vi "ROV Control via UDP Protocole. upgrade.vi"() -> ()   [LabVIEW 2012]
uses:
  <vilib>/Utility/inputDevices.llb/closeJoystick.vi
  <vilib>/Utility/inputDevices.llb/joystickAcquire.vi
panel:
  in  "J":dbl
  out "CASE Z R":u32
  out "CASE UP AND DOWN":u32
  in  "LED STATE":dbl
  in  "N result":string
  out "CASE MOTION":u32
  out "Y O":dbl
  out "U O":dbl
  out "Z O":dbl
  out "X O":dbl
  out "Z R O":dbl
  out "axis info":T1
  out "direction info":T2
  out "button info":T3
  in  "device index":i32
  out "joystick info":T4(array[cluster])
  out "Result":string
  in  "I":dbl
  in  "H":dbl
  in  "G":dbl
  in  "D":dbl
  in  "E":dbl
  in  "Z":dbl
  in  "F":dbl
  in  "C":dbl
  in  "Y":dbl
  in  "B":dbl
  in  "A":dbl
  in  "?":bool
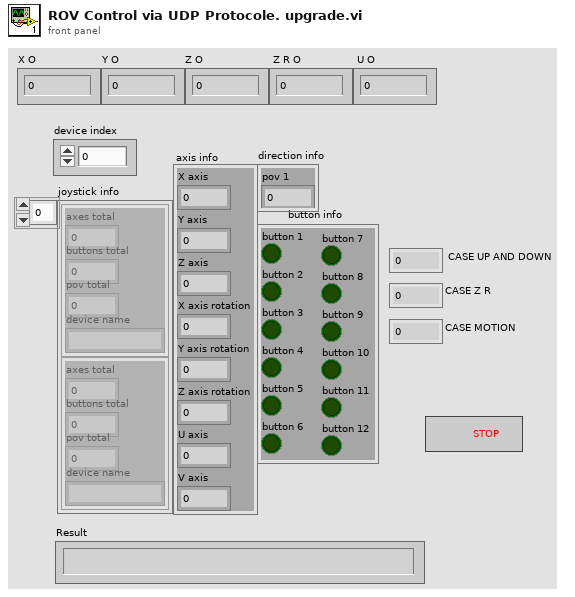
[diagram p1: front panel]
types:
  T1 = cluster{"X axis":i32, "Y axis":i32, "Z axis":i32, "X axis rotation":i32, "Y axis rotation":i32, "Z axis rotation":i32, "U axis":i32, "V axis":i32}
  T2 = cluster{"pov 1":i32, "pov 2":i32, "pov 3":i32, "pov 4":i32}
  T3 = cluster{"button 1":bool, "button 2":bool, "button 3":bool, "button 4":bool, "button 5":bool, "button 6":bool, "button 7":bool, "button 8":bool, "button 9":bool, "button 10":bool, "button 11":bool, "button 12":bool, "button 13":bool, "button 14":bool, "button 15":bool, "button 16":bool, "button 17":bool, "button 18":bool, "button 19":bool, "button 20":bool, "button 21":bool, "button 22":bool, "button 23":bool, "button 24":bool, "button 25":bool, "button 26":bool, "button 27":bool, "button 28":bool, "button 29":bool, "button 30":bool, "button 31":bool, "button 32":bool}
  T4 = cluster{"axes total":u32, "buttons total":u32, "pov total":u32, "device name":string}[]
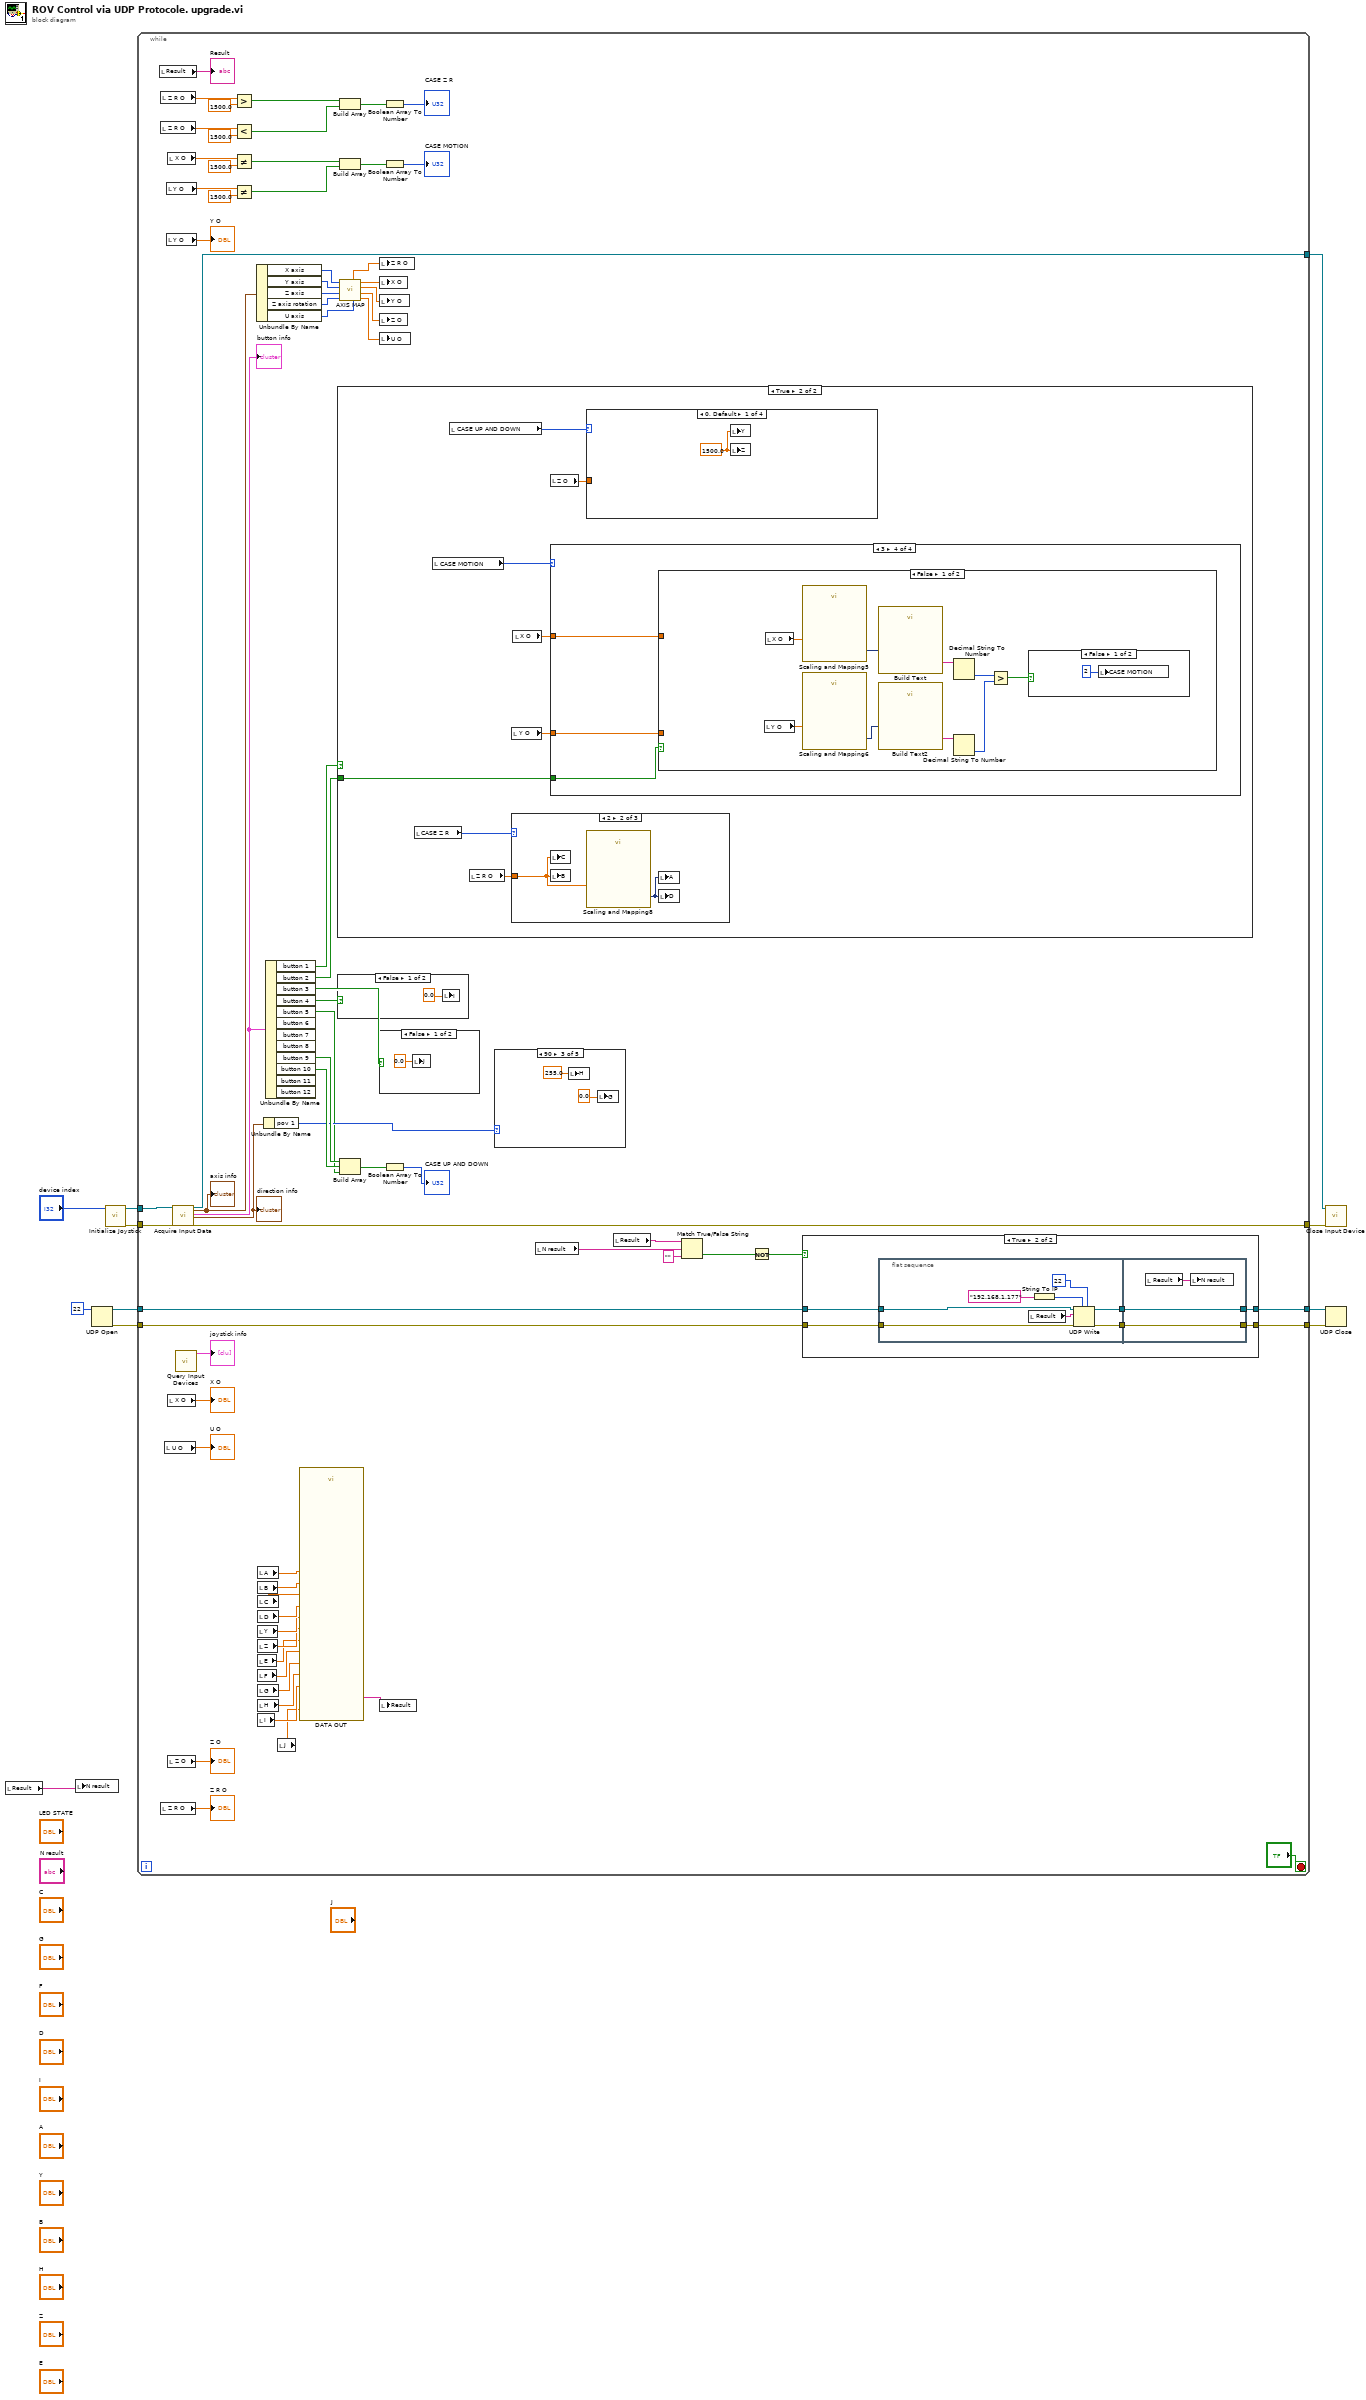
[diagram p0: block diagram]
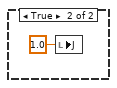
[diagram p2: hidden frame]
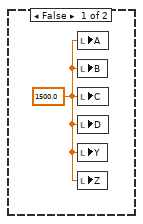
[diagram p3: hidden frame]
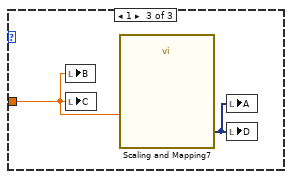
[diagram p5: hidden frame]
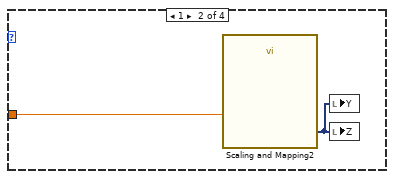
[diagram p6: hidden frame]
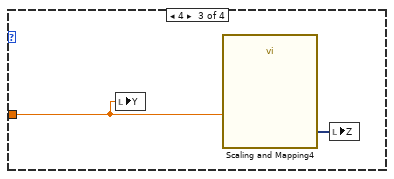
[diagram p7: hidden frame]
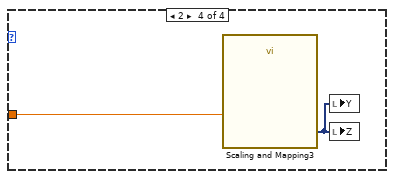
[diagram p8: hidden frame]
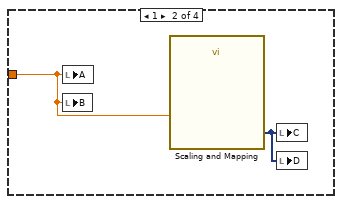
[diagram p10: hidden frame]
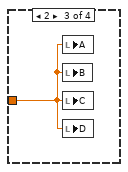
[diagram p11: hidden frame]
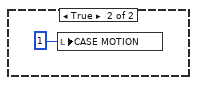
[diagram p12: hidden frame]
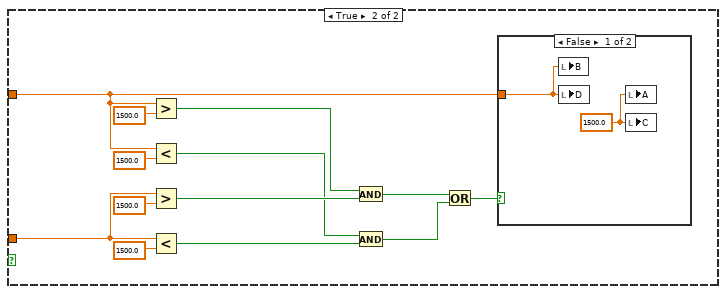
[diagram p13: hidden frame]
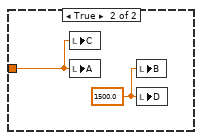
[diagram p14: hidden frame]
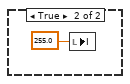
[diagram p15: hidden frame]
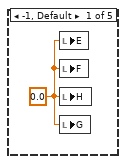
[diagram p17: hidden frame]
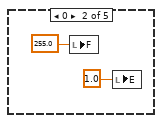
[diagram p18: hidden frame]
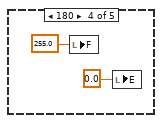
[diagram p19: hidden frame]
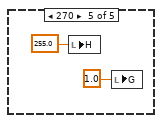
[diagram p20: hidden frame]
diagram:
  n1 = local read "Result"() -> (w1:string)
  n2 = local write "N result"(w1) -> ()
  n3 = UDP Open(11:u16 22 ("port")) -> (port=w5:refnum<k16>, 0:w4:errorcluster)  [unwired: 4 in, 1 out]
  n4 = call <vilib>:"Initialize Joystick.vi"("device index"="device index") -> ("error out"=w10:errorcluster, "device ID"=w11:refnum<k1>)  [unwired: 9 in]
  n5 = while {
    tunnel: w11 -> [w70]
    tunnel: w10 -> [w69]
    tunnel: [w68] -> w9
    tunnel: [w67] -> w8
    tunnel: w5 -> [w28]
    tunnel: w4 -> [w29]
    tunnel: [w27] -> w3
    tunnel: [w26] -> w2
    stop <- "?" stop-if-true
    n6 = local read "Result"() -> (→"Result":string)
    n7 = local read "Z R O"() -> (w21:dbl)
    n8 = local read "Z R O"() -> (w19:dbl)
    n9 = local read "Z R O"() -> (→"Z R O":dbl)
    n10 = local read "U O"() -> (→"U O":dbl)
    n11 = local read "Y O"() -> (w46:dbl)
    n12 = local read "Y O"() -> (→"Y O":dbl)
    n13 = local read "X O"() -> (w47:dbl)
    n14 = local read "X O"() -> (→"X O":dbl)
    n15 = local read "Z O"() -> (→"Z O":dbl)
    n16 = call-poly <vilib>:"Acquire Input Data.vi"("device ID"=w70, "error in (no error)"=w69) -> ("device ID"=w68:refnum<k1>, "axis info"=w63:T1, "button info"=w65:T3, "direction info"=w64:T2, "error out"=w67:errorcluster)  [unwired: 13 in]
    "button info" <- w65
    "direction info" <- w64
    "axis info" <- w63
    n17 = call <vilib>:"Query Input Devices.vi"() -> ("joystick info"=→"joystick info":T4)  [unwired: 8 in, 3 out]
    n18 = Greater?(x=w21, y=1500.0) -> (0:w23:bool)
    n19 = Less?(x=w19, y=1500.0) -> (x < y?=w17:bool)
    n20 = Not Equal?(x=w47, y=1500.0) -> (x != y?=w43:bool)
    n21 = Not Equal?(x=w46, y=1500.0) -> (x != y?=w42:bool)
    n22 = Unbundle By Name(w63) -> ("X axis"=w62:i32, "Y axis"=w61:i32, "Z axis"=w60:i32, "Z axis rotation"=w59:i32, "U axis"=w58:i32)
    n23 = local read "A"() -> (w83:dbl)
    n24 = local read "B"() -> (w82:dbl)
    n25 = local read "C"() -> (w81:dbl)
    n26 = local read "D"() -> (w80:dbl)
    n27 = local read "Y"() -> (w79:dbl)
    n28 = local read "Z"() -> (w78:dbl)
    n29 = local read "E"() -> (w77:dbl)
    n30 = local read "F"() -> (w76:dbl)
    n31 = local read "G"() -> (w75:dbl)
    n32 = local read "H"() -> (w74:dbl)
    n33 = local read "I"() -> (w73:dbl)
    n34 = Unbundle By Name(w64) -> ("pov 1"=w35:i32)
    n35 = Unbundle By Name(w65) -> ("button 1"=w14:bool, "button 2"=w15:bool, "button 3"=w12:bool, "button 4"=w25:bool, "button 5"=w24:bool, "button 9"=w39:bool, "button 10"=w38:bool)  [unwired: 5 out]
    n36 = local read "J"() -> (w13:dbl)
    n37 = call "DATA OUT"("a"=w83, "b"=w82, "c"=w81, "d"=w80, "y"=w79, "z"=w78, "e"=w77, "f"=w76, "g"=w75, "h"=w74, "i"=w73, "j"=w13) -> ("Result"=w72:string)  [unwired: 14 in, 1 out]
    n38 = case shown="True" w14 {
      tunnel: w15 -> [_ w90]
      frame False {
        w87 = 1500.0 ("B")
        n39 = local write "A"(w87) -> ()
        n40 = local write "B"(w87) -> ()
        n41 = local write "C"(w87) -> ()
        n42 = local write "D"(w87) -> ()
        n43 = local write "Y"(w87) -> ()
        n44 = local write "Z"(w87) -> ()
      }
      frame True {
        n45 = local read "CASE Z R"() -> (w89:u32)
        n46 = local read "CASE MOTION"() -> (w92:u32)
        n47 = local read "CASE UP AND DOWN"() -> (w88:u32)
        n48 = local read "Z R O"() -> (w91:dbl)
        n49 = local read "Y O"() -> (w94:dbl)
        n50 = case shown="2" w89 {
          tunnel: w91 -> [_ w96 w99]
          frame 0, Default {
          }
          frame 2 {
            n51 = local write "C"(w96) -> ()
            n52 = local write "B"(w96) -> ()
            n53 = call "Scaling and Mapping8"("Signals"=w96) -> ("Scaled Signals"=w97:dynamicdata)  [unwired: 9 in, 1 out]
            n54 = local write "A"(w97) -> ()
            n55 = local write "D"(w97) -> ()
          }
          frame 1 {
            n56 = local write "B"(w99) -> ()
            n57 = local write "C"(w99) -> ()
            n58 = call "Scaling and Mapping7"("Signals"=w99) -> ("Scaled Signals"=w98:dynamicdata)  [unwired: 9 in, 1 out]
            n59 = local write "A"(w98) -> ()
            n60 = local write "D"(w98) -> ()
          }
        }
        n61 = local read "X O"() -> (w95:dbl)
        n62 = local read "Z O"() -> (w93:dbl)
        n63 = case shown="3" w92 {
          tunnel: w95 -> [_ w108 _ w111]
          tunnel: w94 -> [_ _ w109 w112]
          tunnel: w90 -> [_ _ _ w110]
          frame 0, Default {
          }
          frame 1 {
            n64 = local write "A"(w108) -> ()
            n65 = local write "B"(w108) -> ()
            n66 = call "Scaling and Mapping"("Signals"=w108) -> ("Scaled Signals"=w107:dynamicdata)  [unwired: 9 in, 1 out]
            n67 = local write "C"(w107) -> ()
            n68 = local write "D"(w107) -> ()
          }
          frame 2 {
            n69 = local write "A"(w109) -> ()
            n70 = local write "B"(w109) -> ()
            n71 = local write "C"(w109) -> ()
            n72 = local write "D"(w109) -> ()
          }
          frame 3 {
            n73 = case shown="False" w110 {
              tunnel: w112 -> [_ w127]
              tunnel: w111 -> [_ w124]
              frame False {
                n74 = local read "Y O"() -> (w120:dbl)
                n75 = local read "X O"() -> (w121:dbl)
                n76 = call "Scaling and Mapping5"("Signals"=w121) -> ("Scaled Signals"=w117:dynamicdata)  [unwired: 9 in, 1 out]
                n77 = call "Scaling and Mapping6"("Signals"=w120) -> ("Scaled Signals"=w115:dynamicdata)  [unwired: 9 in, 1 out]
                n78 = call "Build Text"("Z"=w117) -> ("Result"=w118:string)  [unwired: 13 in, 1 out]
                n79 = call "Build Text2"("Z"=w115) -> ("Result"=w116:string)  [unwired: 13 in, 1 out]
                n80 = Decimal String To Number(string=w118) -> (number=w113:i32)  [unwired: 2 in, 1 out]
                n81 = Decimal String To Number(string=w116) -> (number=w114:i32)  [unwired: 2 in, 1 out]
                n82 = Greater?(x=w113, y=w114) -> (0:w119:bool)
                n83 = case shown="False" w119 {
                  frame False {
                    n84 = local write "CASE MOTION"(u32 2 ("number")) -> ()
                  }
                  frame True {
                    n85 = local write "CASE MOTION"(u32 1 ("number")) -> ()
                  }
                }
              }
              frame True {
                n86 = Greater?(x=w124, y=1500.0) -> (0:w136:bool)
                n87 = Less?(x=w124, y=1500.0) -> (x < y?=w128:bool)
                n88 = Greater?(x=w127, y=1500.0) -> (0:w135:bool)
                n89 = Less?(x=w127, y=1500.0) -> (x < y?=w129:bool)
                n90 = And(x=w136, y=w135) -> (x .and. y?=w132:bool)
                n91 = And(x=w128, y=w129) -> (x .and. y?=w126:bool)
                n92 = Or(x=w132, y=w126) -> (x .or. y?=w125:bool)
                n93 = case shown="False" w125 {
                  tunnel: w124 -> [w138 w140]
                  frame False {
                    w137 = 1500.0 ("D")
                    n94 = local write "B"(w138) -> ()
                    n95 = local write "D"(w138) -> ()
                    n96 = local write "A"(w137) -> ()
                    n97 = local write "C"(w137) -> ()
                  }
                  frame True {
                    w139 = 1500.0 ("B")
                    n98 = local write "C"(w140) -> ()
                    n99 = local write "A"(w140) -> ()
                    n100 = local write "B"(w139) -> ()
                    n101 = local write "D"(w139) -> ()
                  }
                }
              }
            }
          }
        }
        n102 = case shown="0, Default" w88 {
          tunnel: w93 -> [_ w102 w103 w105]
          frame 0, Default {
            w100 = 1500.0 ("Y")
            n103 = local write "Y"(w100) -> ()
            n104 = local write "Z"(w100) -> ()
          }
          frame 1 {
            n105 = call "Scaling and Mapping2"("Signals"=w102) -> ("Scaled Signals"=w101:dynamicdata)  [unwired: 9 in, 1 out]
            n106 = local write "Y"(w101) -> ()
            n107 = local write "Z"(w101) -> ()
          }
          frame 4 {
            n108 = local write "Y"(w103) -> ()
            n109 = call "Scaling and Mapping4"("Signals"=w103) -> ("Scaled Signals"=w104:dynamicdata)  [unwired: 9 in, 1 out]
            n110 = local write "Z"(w104) -> ()
          }
          frame 2 {
            n111 = call "Scaling and Mapping3"("Signals"=w105) -> ("Scaled Signals"=w106:dynamicdata)  [unwired: 9 in, 1 out]
            n112 = local write "Y"(w106) -> ()
            n113 = local write "Z"(w106) -> ()
          }
        }
      }
    }
    n114 = case shown="False" w25 {
      frame False {
        n115 = local write "I"(0.0 ("I")) -> ()
      }
      frame True {
        n116 = local write "I"(255.0 ("I")) -> ()
      }
    }
    n117 = Build Array(w23, w17) -> (w20:bool[])
    n118 = Build Array(w43, w42) -> (w41:bool[])
    n119 = call "AXIS MAP.vi"("X I"=w62, "Y I"=w61, "Z I"=w60, "Z R I"=w59, "U I"=w58) -> ("Z R O"=w48:dbl, "X O"=w52:dbl, "Y O"=w51:dbl, "Z O"=w50:dbl, "U O"=w49:dbl)
    n120 = Build Array(w39, w38, w24) -> (w37:bool[])
    n121 = case shown="False" w12 {
      frame False {
        n122 = local write "J"(0.0 ("J")) -> ()
      }
      frame True {
        n123 = local write "J"(1.0 ("J")) -> ()
      }
    }
    n124 = local write "Z R O"(w48) -> ()
    n125 = local write "X O"(w52) -> ()
    n126 = local write "Y O"(w51) -> ()
    n127 = local write "Z O"(w50) -> ()
    n128 = local write "U O"(w49) -> ()
    n129 = local write "Result"(w72) -> ()
    n130 = Boolean Array To Number(Boolean array=w20) -> (number=→"CASE Z R":u32)
    n131 = Boolean Array To Number(Boolean array=w41) -> (number=→"CASE MOTION":u32)
    n132 = Boolean Array To Number(Boolean array=w37) -> (number=→"CASE UP AND DOWN":u32)
    n133 = case shown="90" w35 {
      frame -1, Default {
        w162 = 0.0 ("F")
        n134 = local write "E"(w162) -> ()
        n135 = local write "F"(w162) -> ()
        n136 = local write "H"(w162) -> ()
        n137 = local write "G"(w162) -> ()
      }
      frame 0 {
        n138 = local write "F"(255.0 ("F")) -> ()
        n139 = local write "E"(1.0 ("H")) -> ()
      }
      frame 90 {
        n140 = local write "H"(255.0 ("E")) -> ()
        n141 = local write "G"(0.0 ("G")) -> ()
      }
      frame 180 {
        n142 = local write "F"(255.0 ("E")) -> ()
        n143 = local write "E"(0.0 ("H")) -> ()
      }
      frame 270 {
        n144 = local write "H"(255.0 ("E")) -> ()
        n145 = local write "G"(1.0 ("G")) -> ()
      }
    }
    n146 = local read "N result"() -> (w32:string)
    n147 = local read "Result"() -> (w31:string)
    n148 = Match True/False String(2:"" ("false string"), 3:w32, 4:w31) -> (0:w34:bool)  [unwired: 1 out]
    n149 = Not(x=w34) -> (.not. x?=w30:bool)
    n150 = case shown="True" w30 {
      tunnel: [w144 w150] -> w27
      tunnel: [w143 w149] -> w26
      tunnel: w28 -> [w144 w145]
      tunnel: w29 -> [w143 w148]
      frame False {
      }
      frame True {
        n151 = flat-sequence {
          tunnel: w145 -> [w152]
          tunnel: w148 -> [w151]
          tunnel: [w154] -> w147
          tunnel: [w153] -> w146
          tunnel: [w160] -> w149
          tunnel: [w161] -> w150
          tunnel: w147 -> [w161]
          tunnel: w146 -> [w160]
          frame #0 {
            n152 = local read "Result"() -> (w158:string)
            n153 = String To IP(1:"192.168.1.177" ("name")) -> (0:w156:u32)
            n154 = UDP Write(address=w156, port or service name=u16 22, connection ID=w152, data in=w158, 8:w151) -> (error out=w153:errorcluster, 3:w154:refnum<k16>)  [unwired: 1 in]
          }
          frame #1 {
            n155 = local read "Result"() -> (w159:string)
            n156 = local write "N result"(w159) -> ()
          }
        }
      }
    }
  }
  n157 = call-poly <vilib>:"Close Input Device.vi"("error in (no error)"=w8, "device ID"=w9) -> ()  [unwired: 8 in, 1 out]
  n158 = UDP Close(connection ID=w3, 8:w2) -> ()  [unwired: 2 out]
